vi "update hydrolysis inflow.vi"(8 "error in (no error)":errorcluster, 9 "fraction":dbl, 10 "hydrolysis_specfile":string, 11 "outflow_infile":string) -> (0 "error out":errorcluster)   [LabVIEW 2019, in "libFileFunctions.lvlib"]
doc: "void update_hydrolysis_inflow(const char* outflow_infile, const char* hydrolysis_specfiles, double fractions[]);"
uses:
  libFileFunctions.lvlib
panel:
  out "fraction out":dbl
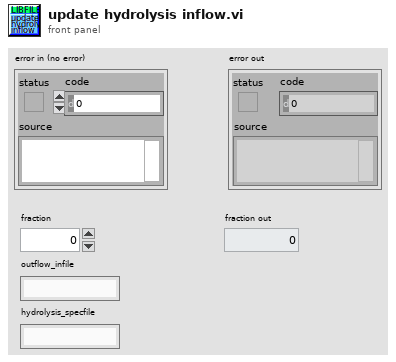
[diagram p1: front panel]
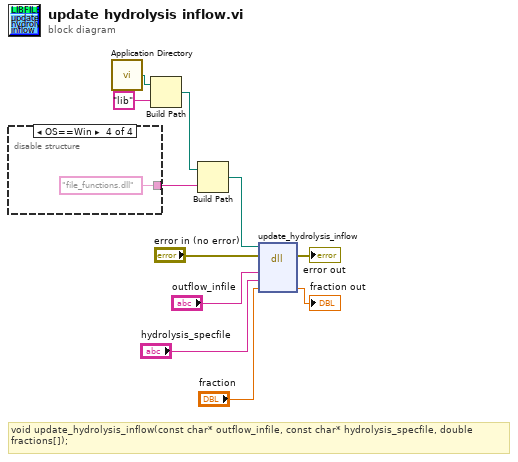
[diagram p0: block diagram]
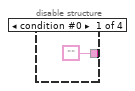
[diagram p2: hidden frame]
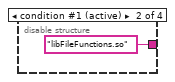
[diagram p3: hidden frame]
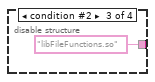
[diagram p4: hidden frame]
diagram:
  # "void update_hydrolysis_inflow(const char* outflow_infile, const char* hydrolysis_specfile, double fractions[]);"
  n1 = disable-structure shown="OS==Win" {
    disable-tunnel: ["" "libFileFunctions.so" ("name or relative path") "libFileFunctions.so" ("name or relative path") "file_functions.dll" ("name or relative path")] -> w5
    frame condition #0 {
    }
    frame condition #1 (active) {
    }
    frame condition #2 {
    }
    frame condition #3 {
    }
  }
  n2 = call <vilib>:"Application Directory.vi"() -> ("Application Directory"=w8:path)
  n3 = Build Path(base path=w8, name or relative path="lib") -> (appended path=w6:path)
  n4 = Build Path(base path=w6, name or relative path=w5) -> (appended path=w4:path)
  n5 = dll-call lib="home/paul/Schreibtisch/Biogas_plant_setup/LabView/lib/libFileFunctions/libFileFunctions.*" fn="update_hydrolysis_inflow"(path in=w4, error in="error in (no error)", "outflow_infile"="outflow_infile", "hydrolysis_specfile"="hydrolysis_specfile", "fraction"="fraction") -> (error out=→"error out":errorcluster, "fraction"=→"fraction out":dbl)  [unwired: 4 in, 1 out]
